vi "Send Set Letter Time.vi"(7 "Message Priority (Normal)":T1=enum."Normal", 8 "error in (no error)":errorcluster, 9 "Time":dbl[unit], 10 "Letter":string, 11 "Message Enqueuer":refnum<class "Message Enqueuer.lvclass">) -> (0 "error out":errorcluster, 3 "Message Enqueuer out":refnum<class "Message Enqueuer.lvclass">)   [LabVIEW 2016, in "CS++PPG.lvlib" / "Set Letter Time Msg.lvclass"]
doc: "Sends the <B>CS++PPG.lvlib:Set Letter Time Msg.lvclass</B> message.\n\n<B>CS++PPG.lvlib:CS++PPG.lvclass:Set Letter Time.vi</B> Description:\n\nThis VI sets a new time value for a given letter of the timing pattern. This should also work while the pulsed pattern generator is running."
uses:
  Set Letter Time Msg.lvclass
  <vilib>/ActorFramework/Message Enqueuer/Message Enqueuer.lvclass
  <vilib>/ActorFramework/Message Enqueuer/Message Priority.ctl
  C:/Program Files (x86)/National Instruments/LabVIEW 2016/vi.lib/ActorFramework/Message/Message.lvclass
  Set Letter Time Msg.lvclass/Set Letter Time Msg.ctl
  <vilib>/ActorFramework/Message Enqueuer/Message Enqueuer.lvclass/Message Enqueuer.ctl
  <vilib>/ActorFramework/Message Priority Queue/Priority Enqueue.vi
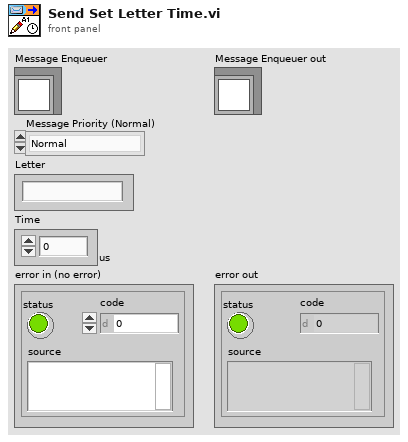
[diagram p1: front panel]
types:
  T1 = typedef "Actor Framework.lvlib/Message Enqueuer.lvclass/Message Priority.ctl" = enum16{"Low", "Normal", "High"}
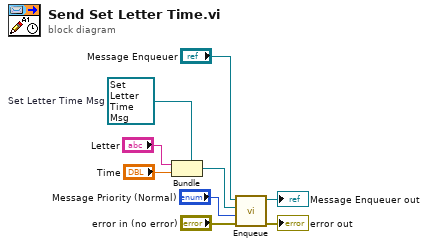
[diagram p0: block diagram]
diagram:
  w3 = refnum<class "Set Letter Time Msg.lvclass"> refnum  # Set Letter Time Msg
  n1 = Bundle(cluster=w3, "Letter", "Time") -> (w6:refnum<class "Set Letter Time Msg.lvclass">)
  n2 = call <vilib>:"Enqueue.vi"("error in (no error)"="error in (no error)", "Message Priority (Normal)"="Message Priority (Normal)", "Message"=w6, "Message Enqueuer in"="Message Enqueuer") -> ("error out"=→"error out":errorcluster, "Message Enqueuer out"=→"Message Enqueuer out":refnum<class "Message Enqueuer.lvclass">)  [unwired: 6 in]
